vi "modbus2.1.vi"() -> ()   [LabVIEW 2019]
uses:
  <vilib>/MakerHub/LINX/Public/Peripherals/Digital/Digital Write 1 Chan.vi
  <vilib>/MakerHub/LINX/Public/Peripherals/Digital/Digital Write N Chans.vi
  <vilib>/MakerHub/LINX/Private/Local IO/LinxDigitalWrite.vi
  <vilib>/MakerHub/LINX/Public/Utilities/Check Channel.vi
  <vilib>/Modbus/master/Create Master Instance (Serial).vi
  <vilib>/MakerHub/LINX/Public/Utilities/Open Serial.vi
  <vilib>/MakerHub/LINX/Private/Utilties/Generate Error.vi
  <vilib>/Modbus/master/Modbus Master.lvclass
  <vilib>/MakerHub/LINX/LMH-LINX.lvlib
panel:
  in  "Tab Control":enum32{"Main", "Conexão"}(tab)
  out "Motor 2":bool
  in  "Motor":bool
  out "Frequência (Hz)":sgl format="%#_2f"
  in  "x 2":dbl=3.0 min=3.0 max=60.0 step=1.0
  out "Ciclos 2":sgl caption="Elapsed Time (s)" format="%#_6f"
  in  "Ciclos":sgl=5.0 format="%#_6f"
  in  "Ciclo Ar (s)":dbl
  out "Ciclos encerrados":bool
  out "Injetando ar":bool caption="Time has Elapsed"
  out "Motor 3":bool
  in  "Ar":bool
  in  "stop":bool
  in  "Porta COM":refnum<visa-resource-name>
  in  "baud rate":u32=9600
  in  "parity":u16(ring)=2 items=["None", "Odd", "Even"]
  in  "Porta COM":refnum<visa-resource-name>
  in  "baud rate":u32=9600
  # "Motor"
  # "Ar comprimido"
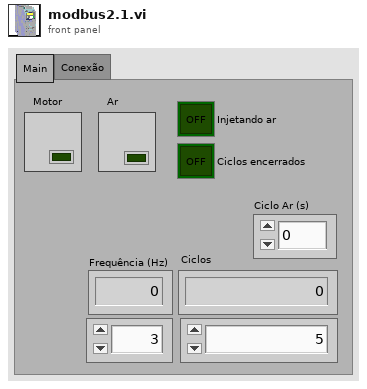
[diagram p1: front panel]
types:
  T1 = typedef "LMH-LINX.lvlib/LINX Ref.ctl" = cluster{"IO":T2, "Interface":T3, "LINX Device Config":T4}
  T2 = typedef "LMH-LINX.lvlib/Platform.ctl" = enum16{"Remote", "Local"}
  T3 = typedef "LMH-LINX.lvlib/Interface.ctl" = enum16{"Serial", "TCP"}
  T4 = typedef "LMH-LINX.lvlib/Device.lvlib/LINX Device Config.ctl" = cluster{"Interface":T3, "COM Port":refnum<visa-resource-name>, "TCP Configuration":T5, "Device Family":u8, "Device ID":u8, "Device Name":string, "TCP Ref":refnum<k5>, "Channels":T6}
  T5 = typedef "LMH-LINX.lvlib/Device.lvlib/TCP Config.ctl" = cluster{"IP Address":string, "Port":u16}
  T6 = typedef "LMH-LINX.lvlib/Channels.ctl" = cluster{"DI":u8[], "DO":u8[], "AI":u8[], "AO":u8[], "PWM":u8[], "QE":u8[], "UART":u8[], "I2C 2":u8[], "SPI":u8[], "CAN":u8[], "Servo":u8[], "AI Ref (V)":dbl, "AI Resolution (Bits)":u8, "AO Ref (V)":dbl, "AO Resolution (Bits)":u8}
  T7 = cluster{"register values[0]":u16, "register values[1]":u16, "register values[2]":u16, "register values[3]":u16, "register values[4]":u16, "register values[5]":u16, "register values[6]":u16, "register values[7]":u16, "register values[8]":u16}
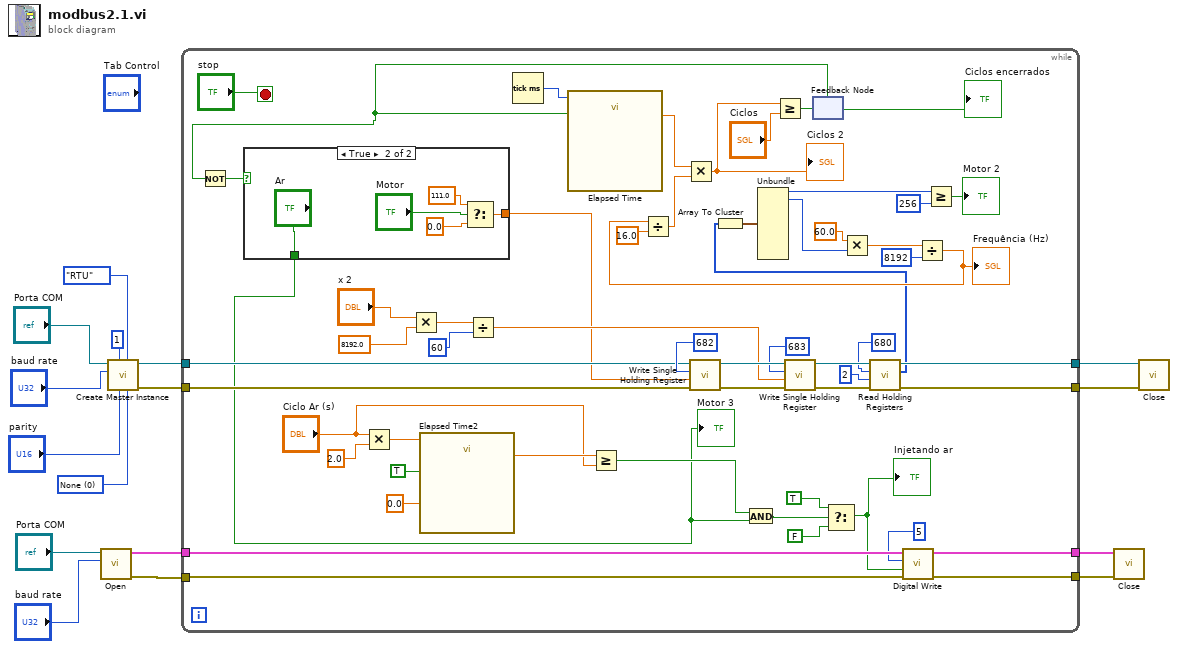
[diagram p0: block diagram]
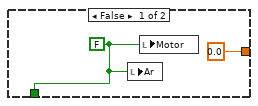
[diagram p2: hidden frame]
diagram:
  w16 = u16 0 items=["None", "XON/XOFF", "RTS/CTS", "XON/XOFF & RTS/CTS", "DTR/DSR", "XON/XOFF & DTR/DSR"] ("flow control (None)")
  n1 = call-poly <vilib>:"Open.vi"("Baud Rate Override"="baud rate", "Serial Port"="Porta COM") -> ("Error Out"=w3:errorcluster, "LINX Resource"=w4:T1)  [unwired: 7 in, 1 out]
  n2 = call-poly <vilib>:"Create Master Instance.vi"("flow control (None)"=w16, "serial type"=enum16{"RTU", "ASCII"}."RTU", "parity (Even)"="parity", "unit ID"=u8 1, "baud rate (9600)"="baud rate", "VISA resource name"="Porta COM") -> ("error out"=w9:errorcluster, "serial master instance"=w10:refnum<class "Modbus Master.lvclass">)  [unwired: 4 in]
  n3 = while {
    tunnel: w10 -> [w65]
    tunnel: w9 -> [w67]
    tunnel: [w61] -> w8
    tunnel: [w60] -> w7
    tunnel: w4 -> [w38]
    tunnel: w3 -> [w37]
    tunnel: [w35] -> w2
    tunnel: [w34] -> w1
    stop <- "stop" stop-if-true
    n4 = Multiply(x="Ciclo Ar (s)", y=2.0) -> (x*y=w25:dbl)
    n5 = Multiply(x="x 2", y=8192.0) -> (x*y=w51:dbl)
    n6 = call "Elapsed Time2"("Time Target (s)"=w25, "Auto Reset"=TRUE, "Set Start Time (s)"=0.0) -> ("Elapsed Time (s)"=w28:dbl)  [unwired: 9 in, 7 out]
    n7 = Divide(x=w51, y=u16 60) -> (x/y=w58:dbl)
    n8 = Tick Count (ms)() -> (millisecond timer value=w48:u32)
    n9 = Greater Or Equal?(x=w28, y="Ciclo Ar (s)") -> (x >= y?=w27:bool)
    n10 = feedback #1() -> (w39:bool)  [unwired: 1 in]
    "Ciclos encerrados" <- w39
    n11 = Not(x=w39) -> (.not. x?=w40:bool)
    n12 = case shown="True" w40 {
      tunnel: [0.0 ("f") w76] -> w33
      tunnel: [w72 "Ar"] -> w18
      frame False {
        w72 = FALSE ("On/Off 2")
        n13 = local write "Ar"(w72) -> ()
        n14 = local write "Motor"(w72) -> ()
      }
      frame True {
        n15 = Select(t=111.0, s="Motor", f=0.0) -> (s? t:f=w76:dbl)
      }
    }
    "Motor 3" <- w18
    n16 = call "Elapsed Time"("Time Target (s)"=w48, "Reset"=w39) -> ("Elapsed Time (s)"=w32:dbl)  [unwired: 10 in, 7 out]
    n17 = call-dynamic "Write Single Holding Register.vi"("error in (no error)"=w67, "holding register value"=w33, "address"=u16 682 ("starting address"), "Modbus master in"=w65) -> ("error out"=w68:errorcluster, "Modbus master out"=w69:refnum<class "Modbus Master.lvclass">)  [unwired: 6 in]
    n18 = And(x=w27, y=w18) -> (x .and. y?=w19:bool)
    n19 = call-dynamic "Write Single Holding Register.vi"("error in (no error)"=w68, "holding register value"=w58, "address"=u16 683 ("starting address"), "Modbus master in"=w69) -> ("error out"=w70:errorcluster, "Modbus master out"=w71:refnum<class "Modbus Master.lvclass">)  [unwired: 6 in]
    n20 = Select(t=TRUE, s=w19, f=FALSE) -> (s? t:f=w17:bool)
    "Injetando ar" <- w17
    n21 = call-dynamic "Read Holding Registers.vi"("error in (no error)"=w70, "number of holding registers"=u16 2, "starting address"=u16 680, "Modbus master in"=w71) -> ("error out"=w61:errorcluster, "register values"=w22:u16[], "Modbus master out"=w60:refnum<class "Modbus Master.lvclass">)  [unwired: 5 in]
    n22 = Array To Cluster(array=w22) -> (cluster=w44:T7)
    n23 = Unbundle(w44) -> ("register values[0]"=w21:u16, "register values[1]"=w20:u16)  [unwired: 7 out]
    n24 = Multiply(x=60.0, y=w20) -> (x*y=w57:dbl)
    n25 = call-poly <vilib>:"Digital Write.vi"("Error In"=w37, "Output Value"=w17, "DO Channel"=u8 5, "LINX Resource"=w38) -> ("Error Out"=w35:errorcluster, "LINX Resource"=w34:T1)  [unwired: 6 in]
    n26 = Divide(x=w57, y=u16 8192) -> (x/y=w42:dbl)
    "Frequência (Hz)" <- w42
    n27 = Divide(x=w42, y=16.0) -> (x/y=w47:dbl)
    n28 = Multiply(x=w32, y=w47) -> (x*y=w41:dbl)
    "Ciclos 2" <- w41
    n29 = Greater Or Equal?(x=w41, y="Ciclos") -> (x >= y?=w45:bool)
    n30 = feedback-in #1(w45) -> ()
    n31 = Greater Or Equal?(x=w21, y=u16 256) -> (x >= y?=→"Motor 2":bool)
  }
  n32 = call <vilib>:"Close.vi"("Error In"=w2, "LINX Resource"=w1) -> ()  [unwired: 9 in, 1 out]
  n33 = call-dynamic <vilib>:"Close.vi"("error in (no error)"=w8, "Modbus master in"=w7) -> ()  [unwired: 9 in, 1 out]
